vi "R5ShutDown.vi"() -> ()   [LabVIEW 2016]
panel:
  out "R1SBR_Manual":T1
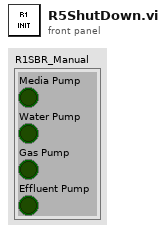
[diagram p1: front panel]
types:
  T1 = cluster{"Media Pump":bool, "Water Pump":bool, "Gas Pump":bool, "Effluent Pump":bool}
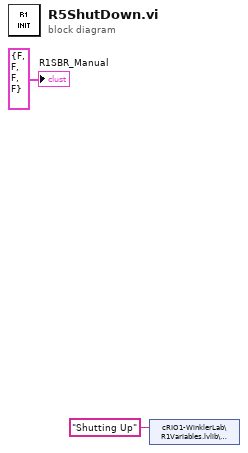
[diagram p0: block diagram]
diagram:
  n1 = shared-variable "cRIO1-WinklerLab\\R1Variables.lvlib\\R1Status"("Shutting Up" ("R1Status")) -> ()  [unwired: 1 in, 1 out]
  "R1SBR_Manual" <- T1 {"Media Pump"=FALSE, "Water Pump"=FALSE, "Gas Pump"=FALSE, "Effluent Pump"=FALSE} ("R1SBR_Manual")
